vi "Add Result Channels.vi"(8 "error in (no error)":errorcluster, 9 "Selected Source Waveform items":T1[](array[typedef]) format="%.0x", 10 "Selected Waveform Section items":T1[](array[typedef]) format="%.0x", 11 "LatestValueCalculation in":refnum<class "LatestValueCalculation.lvclass">) -> (0 "error out":errorcluster, 3 "LatestValueCalculation out":refnum<class "LatestValueCalculation.lvclass">)   [LabVIEW 2015, in "LatestValueCalculation.lvclass"]
uses:
  Waveform-Processing-Custom-Device Configuration.llb/LatestValueCalculation.lvclass
  Waveform-Processing-Custom-Device Configuration.llb/Custom Device Item Ref.ctl
  Waveform-Processing-Custom-Device Configuration.llb/WaveformCalculation.lvclass/WaveformCalculation.ctl
  Waveform-Processing-Custom-Device Configuration.llb/Custom Device Channel.ctl
  Waveform-Processing-Custom-Device Configuration.llb/Custom Device Channel Type.ctl
  Waveform-Processing-Custom-Device Configuration.llb/WaveformCalculation.lvclass
  Waveform-Processing-Custom-Device Configuration.llb/Custom Device API.lvlib
  Waveform-Processing-Custom-Device Configuration.llb/Waveform-Processing-Custom-Device System Explorer.lvlib
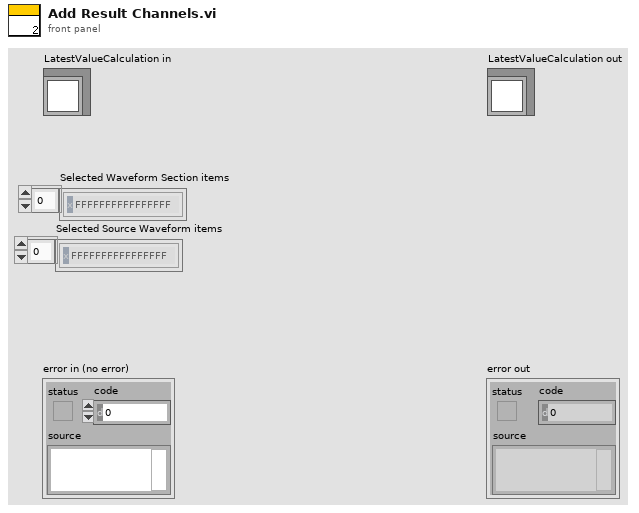
[diagram p1: front panel]
types:
  T1 = typedef "Custom Device API.lvlib/Custom Device Item Ref.ctl" = u64
  T2 = typedef "Custom Device API.lvlib/Custom Device Channel.ctl" = cluster{"Type":T3, "Units":string, "Default Value":dbl, "Faultable":bool, "Scalable":bool}
  T3 = typedef "Custom Device API.lvlib/Custom Device Channel Type.ctl" = enum16{"Input", "Output"}
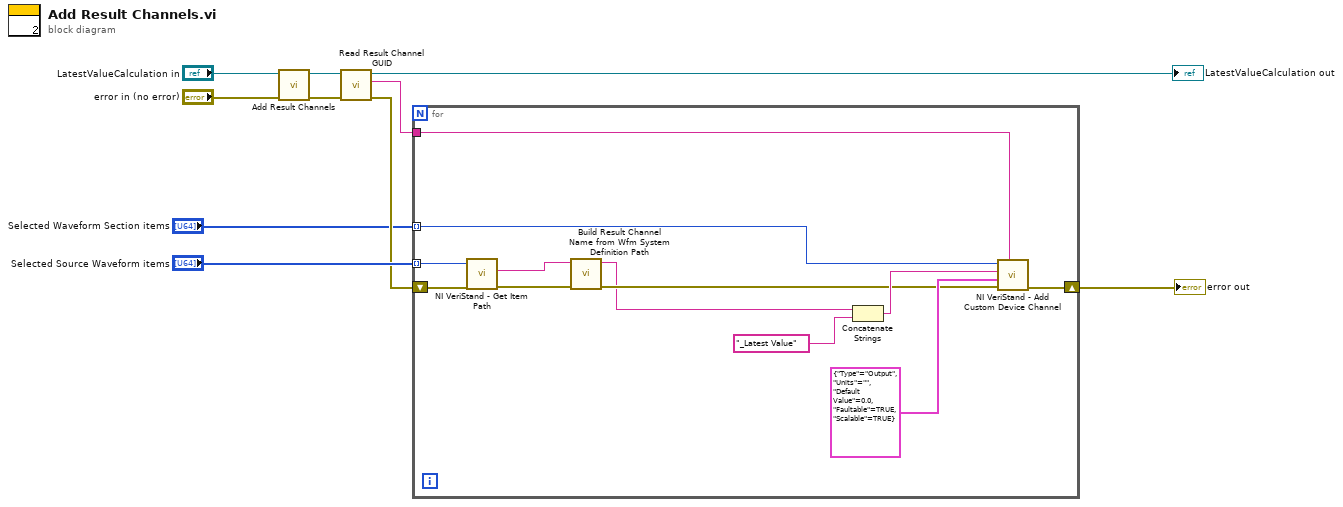
[diagram p0: block diagram]
diagram:
  n1 = call-parent "Add Result Channels.vi"("error in (no error)"="error in (no error)", "WaveformCalculation in"="LatestValueCalculation in") -> ("error out"=w3:errorcluster, "WaveformCalculation out"=w2:refnum<class "LatestValueCalculation.lvclass">)  [unwired: 8 in]
  n2 = call "Read Result Channel GUID.vi"("error in (no error)"=w3, "WaveformCalculation in"=w2) -> ("error out"=w8:errorcluster, "Result Channel GUID"=w9:string, "WaveformCalculation out"=→"LatestValueCalculation out":refnum<class "LatestValueCalculation.lvclass">)  [unwired: 7 in]
  n3 = for {
    tunnel: "Selected Source Waveform items" -> [w16] mode=indexing
    shift-right: [w18] -> w6
    shift-left: w8 -> [w17]
    tunnel: w9 -> [w19]
    tunnel: "Selected Waveform Section items" -> [w11] mode=indexing
    n4 = call "NI VeriStand - Get Item Path.vi"("error in (no error)"=w17, "Item Ref in"=w16) -> ("error out"=w15:errorcluster, "Path"=w13:string)  [unwired: 6 in, 2 out]
    n5 = call "Build Result Channel Name from Wfm System Definition Path.vi"("error in (no error)"=w15, "Channel Path"=w13) -> ("error out"=w14:errorcluster, "delimited string"=w12:string)  [unwired: 8 in]
    n6 = Concatenate Strings(w12, "_Latest Value" ("string")) -> (w21:string)
    n7 = call "NI VeriStand - Add Custom Device Channel.vi"("GUID (Default Channel)"=w19, "error in (no error)"=w14, "Channel"=T2 {"Type"=enum."Output", "Units"="", "Default Value"=0.0, "Faultable"=TRUE, "Scalable"=TRUE}, "Channel Name"=w21, "Parent Ref in"=w11) -> ("error out"=w18:errorcluster)  [unwired: 3 in, 3 out]
  }
  "error out" <- w6
